vi "Metronome_jagther.vi"() -> ()   [LabVIEW 2015]
panel:
  in  "stop":bool
  out "Random Number":dbl
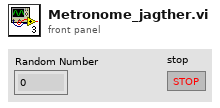
[diagram p1: front panel]
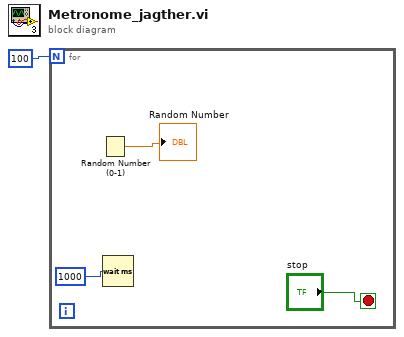
[diagram p0: block diagram]
diagram:
  n1 = for {
    N: 100 -> [_]
    stop <- "stop" stop-if-true
    n2 = Random Number (0-1)() -> (number: 0 to 1=→"Random Number":dbl)
    n3 = Wait (ms)(milliseconds to wait=1000) -> ()  [unwired: 1 out]
  }
